vi "Clear Screen.vi"(10 "Fill colour (Black)":u32(colorbox), 11 "Screen Dimensions":T1) -> (3 "Picture out":picture)   [LabVIEW 2020]
uses:
  Controls/Screen Dimensions.ctl
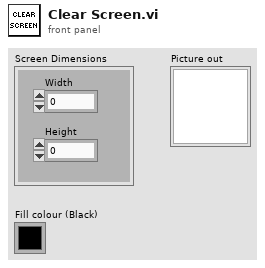
[diagram p1: front panel]
types:
  T1 = typedef "Screen Dimensions.ctl" = cluster{"Width":u32, "Height":u32}
  T2 = cluster{"left":i16, "top":i16, "right":i16, "bottom":i16}
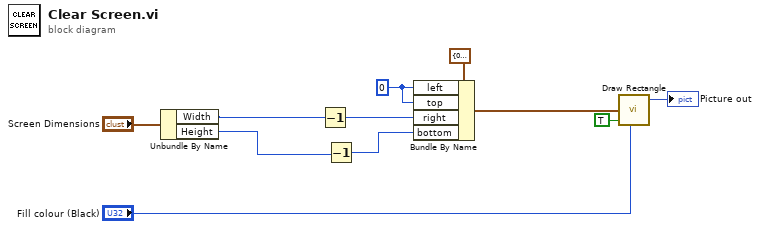
[diagram p0: block diagram]
diagram:
  w2 = i16 0 ("left")
  n1 = Unbundle By Name("Screen Dimensions") -> ("Width"=w9:u32, "Height"=w10:u32)
  n2 = Decrement(x=w9) -> (x-1=w3:u32)
  n3 = Decrement(x=w10) -> (x-1=w4:u32)
  n4 = Bundle By Name(cluster=T2 {"left"=0, "top"=0, "right"=0, "bottom"=0} ("rect"), "left"=w2, "top"=w2, "right"=w3, "bottom"=w4) -> (w5:T2)
  n5 = call <vilib>:"Draw Rectangle.vi"("rect"=w5, "fill?(F)"=TRUE, "color(black)"="Fill colour (Black)") -> ("new picture"=→"Picture out":picture)  [unwired: 6 in]
